vi "AnalyzeHighRateData.vi"(8 "error in (no error)":errorcluster, 9 "data in":T8, 11 "Analysis Configuration In":T1) -> (0 "error out":errorcluster, 1 "data out":T8, 3 "Analysis Configuration Out":T1)   [LabVIEW 2017, in "McsaAnalysisHighRate.lvlib"]
uses:
  <vilib>/addons/InsightCM/Devices/Shared/Mcsa/McsaAnalysisHighRate/McsaAnalysisHighRate.lvlib
  <vilib>/addons/InsightCM/Devices/Shared/Common/DataFlow/controls/Data.ctl
  <vilib>/addons/InsightCM/Utilities/DataAccessors/controls/wfmSGL_DVR.ctl
  <vilib>/addons/PointValueMap/controls/PointMap.ctl
  <vilib>/addons/InsightCM/Devices/Shared/Common/DataFlow/controls/Type.ctl
  <vilib>/addons/InsightCM/Devices/Shared/Mcsa/McsaAnalysisHighRate/controls/Config.ctl
  <vilib>/addons/InsightCM/Devices/Shared/Mcsa/McsaAnalysisHighRate/controls/Group.ctl
  <vilib>/addons/InsightCM/Utilities/Analysis/MCSA/controls/McsaChannel.ctl
  <vilib>/addons/InsightCM/Utilities/Analysis/Shared/controls/Feature.ctl
  <vilib>/addons/InsightCM/Utilities/Analysis/Shared/controls/AmplitudeScale.ctl
  <vilib>/addons/InsightCM/MessageBus/Base/controls/KeyValuePair.ctl
  <vilib>/addons/InsightCM/Utilities/Analysis/MCSA/controls/McsaMotor.ctl
  <vilib>/addons/PointValueMap/PointValueMap.lvlib
  <vilib>/addons/InsightCM/Devices/Shared/Common/DataFlow/DataFlow.lvlib
  <vilib>/addons/InsightCM/Utilities/Analysis/Shared/AnalysisHelper.lvlib
  <vilib>/addons/InsightCM/Utilities/Analysis/MCSA/McsaAnalysisFunctions.lvlib
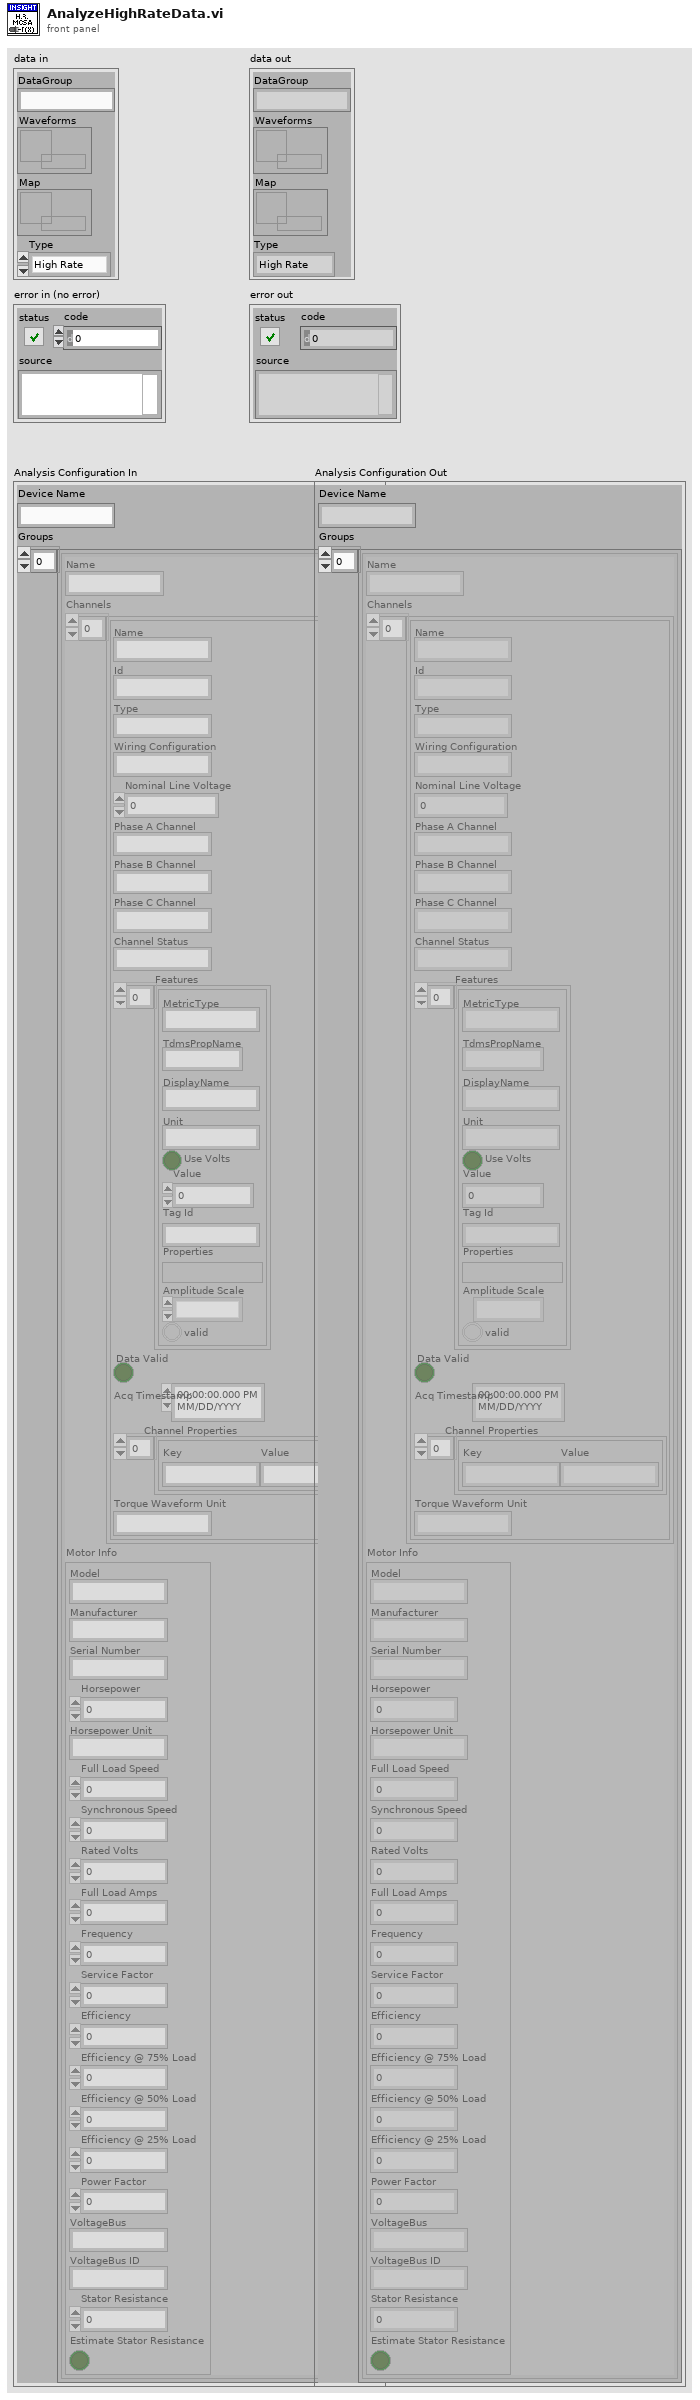
[diagram p1: front panel]
types:
  T1 = typedef "McsaAnalysisHighRate.lvlib/Config.ctl" = cluster{"Device Name":string, "Groups":T2[]}
  T2 = typedef "McsaAnalysisHighRate.lvlib/Group.ctl" = cluster{"Name":string, "Channels":T3[], "Motor Info":T7}
  T3 = typedef "McsaAnalysisFunctions.lvlib/McsaChannel.ctl" = cluster{"Name":string, "Id":string, "Type":string, "Wiring Configuration":string, "Nominal Line Voltage":dbl, "Phase A Channel":string, "Phase B Channel":string, "Phase C Channel":string, "Channel Status":string, "Features":T4[], "Data Valid":bool, "Acq Timestamp":timestamp, "Channel Properties":T6[], "Torque Waveform Unit":string}
  T4 = typedef "AnalysisHelper.lvlib/Feature.ctl" = cluster{"MetricType":string, "TdmsPropName":string, "DisplayName":string, "Unit":string, "Use Volts":bool, "Value":dbl, "Tag Id":string, "Properties":variant, "Amplitude Scale":T5, "valid":bool}
  T5 = typedef "AnalysisHelper.lvlib/AmplitudeScale.ctl" = enum16{"rms", "peak", "pk-pk"}
  T6 = typedef "KeyValuePair.ctl" = cluster{"Key":string, "Value":string}
  T7 = typedef "McsaAnalysisFunctions.lvlib/McsaMotor.ctl" = cluster{"Model":string, "Manufacturer":string, "Serial Number":string, "Horsepower":dbl, "Horsepower Unit":string, "Full Load Speed":dbl, "Synchronous Speed":dbl, "Rated Volts":dbl, "Full Load Amps":dbl, "Frequency":dbl, "Service Factor":dbl, "Efficiency":dbl, "Efficiency @ 75% Load":dbl, "Efficiency @ 50% Load":dbl, "Efficiency @ 25% Load":dbl, "Power Factor":dbl, "VoltageBus":string, "VoltageBus ID":string, "Stator Resistance":dbl, "Estimate Stator Resistance":bool}
  T8 = typedef "DataFlow.lvlib/Data.ctl" = cluster{"DataGroup":string, "Waveforms":T9, "Map":T10, "Type":T11}
  T9 = typedef "wfmSGL_DVR.ctl" = refnum<data-value>
  T10 = typedef "PointValueMap.lvlib/PointMap.ctl" = refnum<data-value>
  T11 = typedef "DataFlow.lvlib/Type.ctl" = enum16{"High Rate", "Low Rate", "Burst Mode"}
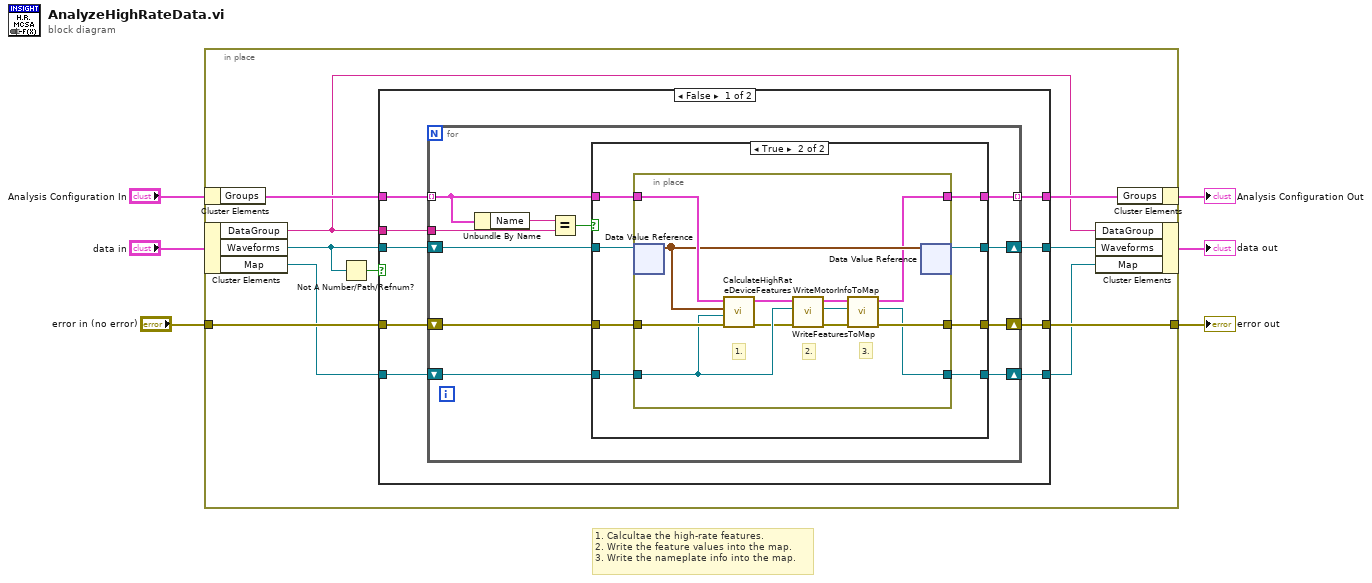
[diagram p0: block diagram]
diagram:
  # "1. Calcultae the high-rate features.\n2. Write the feature values into the map.\n3. Write the nameplate info into the map."
  n1 = in-place {
    in-place-border: [w16] -> w3
    in-place-border: "error in (no error)" -> [w13]
    n2 = in-place-cluster #1("Analysis Configuration In") -> ("Groups"=w15:T2[])
    n3 = in-place-cluster #2("data in") -> ("DataGroup"=w10:string, "Waveforms"=w8:T9, "Map"=w12:T10)
    n4 = Not A Number/Path/Refnum?(number/path/refnum=w8) -> (NaN/Path/Refnum?=w7:bool)
    n5 = case shown="False" w7 {
      tunnel: [w25 w62] -> w16
      tunnel: w15 -> [w24 w64]
      tunnel: [w23 w64] -> w14
      tunnel: w13 -> [w22 w62]
      tunnel: w12 -> [w21 w61]
      tunnel: [w20 w63] -> w11
      tunnel: w10 -> [w19 _]
      tunnel: [w18 w61] -> w9
      tunnel: w8 -> [w17 w63]
      frame False {
        n6 = for {
          tunnel: w19 -> [w33]
          shift-right: [w36] -> w25
          shift-left: w22 -> [w32]
          tunnel: w24 -> [w29] mode=indexing
          tunnel: [w28] -> w23 mode=indexing
          shift-right: [w27] -> w20
          shift-left: w17 -> [w35]
          shift-right: [w26] -> w18
          shift-left: w21 -> [w34]
          n7 = Unbundle By Name(w29) -> ("Name"=w31:string)
          n8 = Equal?(x=w31, y=w33) -> (x = y?=w30:bool)
          n9 = case shown="True" w30 {
            tunnel: [w39 w48] -> w36
            tunnel: w35 -> [w38 w47]
            tunnel: w34 -> [w37 w46]
            tunnel: w32 -> [w39 w45]
            tunnel: w29 -> [w40 w44]
            tunnel: [w40 w43] -> w28
            tunnel: [w38 w42] -> w27
            tunnel: [w37 w41] -> w26
            frame False {
            }
            frame True {
              n10 = in-place {
                in-place-border: w45 -> [w58]
                in-place-border: [w51] -> w48
                in-place-border: [w49] -> w43
                in-place-border: w46 -> [w57]
                in-place-border: w44 -> [w60]
                in-place-border: [w50] -> w41
                # "3."
                # "2."
                # "1."
                n11 = in-place-dvr #3(w47) -> (w59:waveform(sgl)[])  [unwired: 1 out]
                n12 = call <vilib>:"CalculateHighRateDeviceFeatures.vi"("error in (no error)"=w58, "Map in"=w57, "Waveforms"=w59, "Group in"=w60) -> ("error out"=w56:errorcluster, "Group out"=w55:T2)  [unwired: 6 in]
                n13 = call <vilib>:"WriteFeaturesToMap.vi"("error in (no error)"=w56, "Map in"=w57, "Group"=w55) -> ("error out"=w53:errorcluster, "Map out"=w54:T10, "Group out"=w52:T2)  [unwired: 6 in]
                n14 = call <vilib>:"WriteMotorInfoToMap.vi"("error in (no error)"=w53, "Map in"=w54, "Group"=w52) -> ("error out"=w51:errorcluster, "Map out"=w50:T10, "Group out"=w49:T2)  [unwired: 6 in]
                n15 = in-place-dvr #3(w59) -> (w42:T9)  [unwired: 1 out]
              }
            }
          }
        }
      }
      frame True {
      }
    }
    n16 = in-place-cluster #2("DataGroup"=w10, "Waveforms"=w11, "Map"=w9) -> (→"data out":T8)
    n17 = in-place-cluster #1("Groups"=w14) -> (→"Analysis Configuration Out":T1)
  }
  "error out" <- w3
